vi "LV SCISDK Read Oscilloscope.vi"(8 "error in (no error)":errorcluster, 9 "handle":u64, 10 "buffer":T1, 11 "Path":string) -> (0 "error out":errorcluster, 2 "buffer out":T1, 3 "function return":i32)   [LabVIEW 2021, in "SciSDK_Labview.lvlib"]
doc: "SCISDKLABVIEW_DLL_API int LV_SCISDK_ReadOscilloscope(char* Path, TD_OSCILLOSCOPE* buffer, void* handle);"
uses:
  SciSDK_Labview.lvlib
  SciSDK_Labview.dll
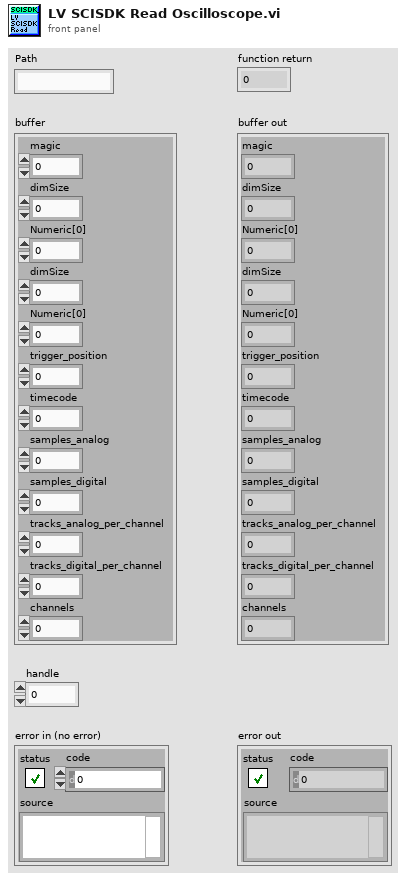
[diagram p1: front panel]
types:
  T1 = cluster{"magic":u32, "dimSize":i32, "Numeric[0]":i32, "dimSize":i32, "Numeric[0]":i32, "trigger_position":u32, "timecode":u32, "samples_analog":u32, "samples_digital":u32, "tracks_analog_per_channel":u32, "tracks_digital_per_channel":u32, "channels":u32}
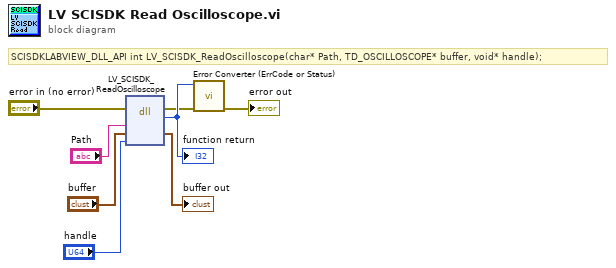
[diagram p0: block diagram]
diagram:
  # "SCISDKLABVIEW_DLL_API int LV_SCISDK_ReadOscilloscope(char* Path, TD_OSCILLOSCOPE* buffer, void* handle);"
  n1 = dll-call lib="C:/git/scisdk/wrapper/LabView/SciSDK_Labview.*" fn="LV_SCISDK_ReadOscilloscope"(error in="error in (no error)", "Path"="Path", "buffer"="buffer", "handle"="handle") -> (error out=w2:errorcluster, w8:i32, "buffer"=→"buffer out":T1)  [unwired: 4 in, 1 out]
  "function return" <- w8
  n2 = call "Error Converter (ErrCode or Status).vi"("error in (no error)"=w2, "error code"=w8) -> ("error out"=→"error out":errorcluster)  [unwired: 9 in]
